vi "util_generate_temp_folder.vi"(8 "error in (no error)":errorcluster) -> (0 "error out":errorcluster, 3 "temp_dir":path)   [LabVIEW 2015, in "lv-build.lvlib"]
uses:
  lv-build.lvlib
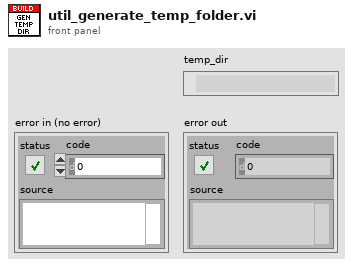
[diagram p1: front panel]
types:
  T1 = typedef "lv-build.lvlib/temp_dir_config.ctl" = cluster{"root_folder":path, "prefix":string}
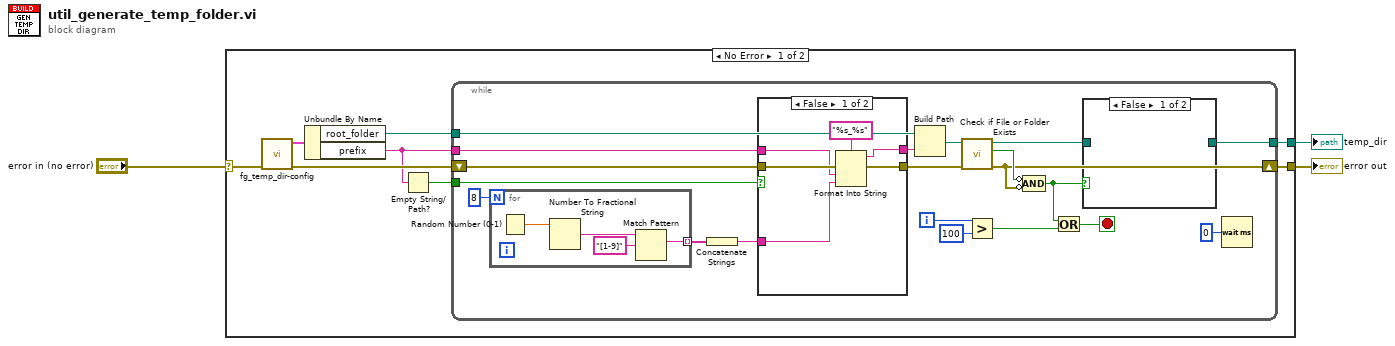
[diagram p0: block diagram]
diagram:
  n1 = case shown="No Error" "error in (no error)" {
    selector: "error in (no error)" -> [w11 w45]
    tunnel: [w5 _] -> w2
    tunnel: [w4 w45] -> w1
    frame No Error {
      n2 = call "fg_temp_dir-config.vi"("error in (no error)"=w11) -> ("error out"=w9:errorcluster, "temp_dir_config"=w10:T1)  [unwired: 9 in]
      n3 = Unbundle By Name(w10) -> ("root_folder"=w8:path, "prefix"=w7:string)
      n4 = Empty String/Path?(string/path=w7) -> (empty?=w6:bool)
      n5 = while {
        tunnel: w7 -> [w28]
        tunnel: w8 -> [w29]
        tunnel: w6 -> [w27]
        shift-right: [w20] -> w4
        shift-left: w9 -> [w26]
        tunnel: [w13] -> w5
        i -> [w18]
        stop <- w19 stop-if-true
        n6 = for {
          N: 8 -> [_]
          tunnel: [w41] -> w31 mode=indexing
          n7 = Random Number (0-1)() -> (number: 0 to 1=w44:dbl)
          n8 = Number To Fractional String(number=w44) -> (F-format string=w43:string)  [unwired: 3 in]
          n9 = Match Pattern(string=w43, regular expression="[1-9]") -> (match substring=w41:string)  [unwired: 1 in, 3 out]
        }
        n10 = Concatenate Strings(w31) -> (w25:string)
        n11 = case shown="False" w27 {
          tunnel: w28 -> [w35 _]
          tunnel: w26 -> [w38 w39]
          tunnel: w25 -> [w34 w40]
          tunnel: [w33 w40] -> w24
          tunnel: [w36 w39] -> w23
          frame False {
            n12 = Format Into String(format string="%s_%s", error in=w38, w35, w34) -> (resulting string=w33:string, error out=w36:errorcluster)  [unwired: 1 in]
          }
          frame True {
          }
        }
        n13 = Build Path(base path=w29, name or relative path=w24) -> (appended path=w22:path)
        n14 = call <vilib>:"Check if File or Folder Exists.vi"("error in (no error)"=w23, "path"=w22) -> ("error out"=w20:errorcluster, "file or folder exists?"=w21:bool, "dup path"=w14:path)  [unwired: 7 in]
        n15 = Greater?(x=w18, y=100) -> (0:w16:bool)
        n16 = Compound Arithmetic op=AND(invert w21, invert w20) -> (w15:bool)
        n17 = Or(x=w15, y=w16) -> (x .or. y?=w19:bool)
        n18 = case shown="False" w15 {
          tunnel: w14 -> [_ w32]
          tunnel: [_ w32] -> w13
          frame False {
          }
          frame True {
          }
        }
        n19 = Wait (ms)(milliseconds to wait=u32 0) -> ()  [unwired: 1 out]
      }
    }
    frame Error {
    }
  }
  "error out" <- w1
  "temp_dir" <- w2
